vi "EX3.vi"() -> ()   [LabVIEW 2018]
panel:
  out "x > y?":bool
  out "Meter":dbl(knob) scale=0.0..30.0 scale format="%#.6g"
  in  "SLIDER CONTROL":dbl(slide) scale=0.0..30.0
  out "date string":string
  out "time string":string
  # "EX3 - TP0"
  # "Mekni Marwen 2ème Année Génie Electrique"
  # "La LED s'allume lorsque le curseur excede la valeur 20"
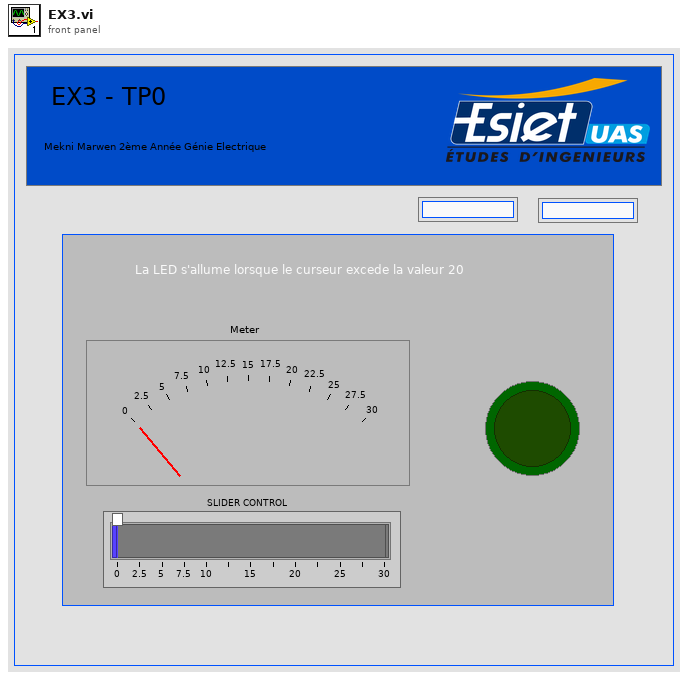
[diagram p1: front panel]
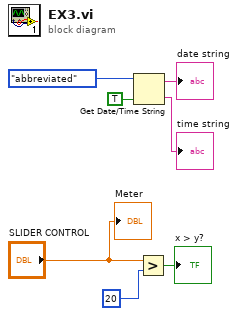
[diagram p0: block diagram]
diagram:
  n1 = Get Date/Time String(date format (0)=enum16{"short", "long", "abbreviated"}."abbreviated", want seconds? (F)=TRUE) -> (date string=→"date string":string, time string=→"time string":string)  [unwired: 1 in]
  n2 = Greater?(x="SLIDER CONTROL", y=20) -> (0:→"x > y?":bool)
  "Meter" <- "SLIDER CONTROL"
